vi "CH_LM ActiveX Control.vi"(0 "Communication Mode":T2, 1 "GPIB Board (0)":i16, 2 "MonitorStop Occurrence":refnum<k4>, 3 "error in (no error)":errorcluster) -> (5 "error out":errorcluster)   [LabVIEW 2017, in "CH_LM.lvlib"]
doc: "This VI is used to register ActiveX Event Callback VIs. Further more a Semaphore is created to make the CH_LM Transaction.vi thread save.\n\nAll important references, ActiveX Control, ActiveX Event Queue and Semaphore are stored in a Fuctional Global Variable for developer access.\n\n<B>Attention:</B> This VI has to be started first and must run all time to monitor event like Meter connected/Disconnected. The communication mode can be selected only once. LabVIEW must be restarted to select another communication mode.\n\n<B>Communication Mode</B> (an enumeration of USB, GPIB, RS232, or None)\nRead/write if no communication channels are open. \nRead only if one or more communication channels are open. \nSpecifies the communication mode. The uninitialized setting will be None. Until this property is set to something other than None:\n\" No events will fire\n\" No I/O activity will take place\n\" The SerialNumber property will return an empty string for any meter index\n\" The SendCommandOrQuery, ConnectToMeter, and DisconnectFromMeter methods will do nothing and return false for any meter index or string argument\n\" The GetNextString method will return an empty string for any meter index"
uses:
  CH_LM.lvlib
  CH_LM Communication Mode.ctl
  _CH_LM/CH_LM Event Cluster.ctl
  _CH_LM/CH_LM Action Enumeration.ctl
  <vilib>/Utility/error.llb/DialogType.ctl
panel:
  out "CH_LM Event Cluster":T1
  in  "CH_LM Event Cluster":T1
  in  "stop":bool
  in  "LM ActiveX Control":refnum<k7>(container)
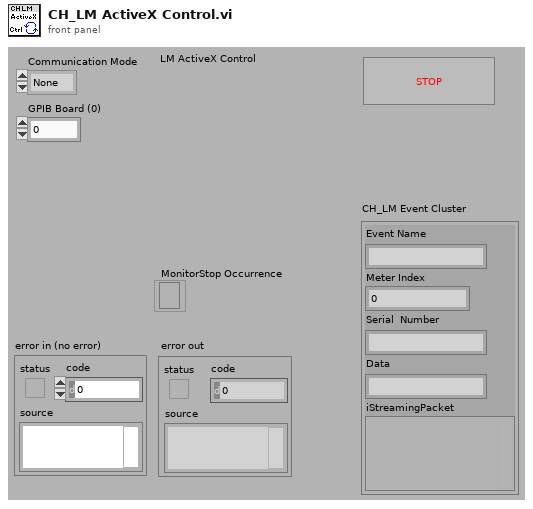
[diagram p1: front panel]
types:
  T1 = typedef "CH_LM.lvlib/CH_LM Event Cluster.ctl" = cluster{"Event Name":string, "Meter Index":i32, "Serial  Number":string, "Data":string, "iStreamingPacket":variant}
  T2 = typedef "CH_LM.lvlib/CH_LM Communication Mode.ctl" = enum16{"None", "USB", "GPIB", "RS232"}
  T3 = typedef "CH_LM.lvlib/CH_LM Action Enumeration.ctl" = enum16{"add", "read", "read by serial", "set", "remove", "delete", "Clear Shift-Register", ""}
  T4 = typedef "Semaphore RefNum" = refnum<k1>
  T5 = typedef "DialogType.ctl" = u16
  T6 = typedef "CH_LM Event Cluster.ctl" = cluster{"Event Name":string, "Meter Index":i32, "Serial  Number":string, "Data":string, "iStreamingPacket":variant}
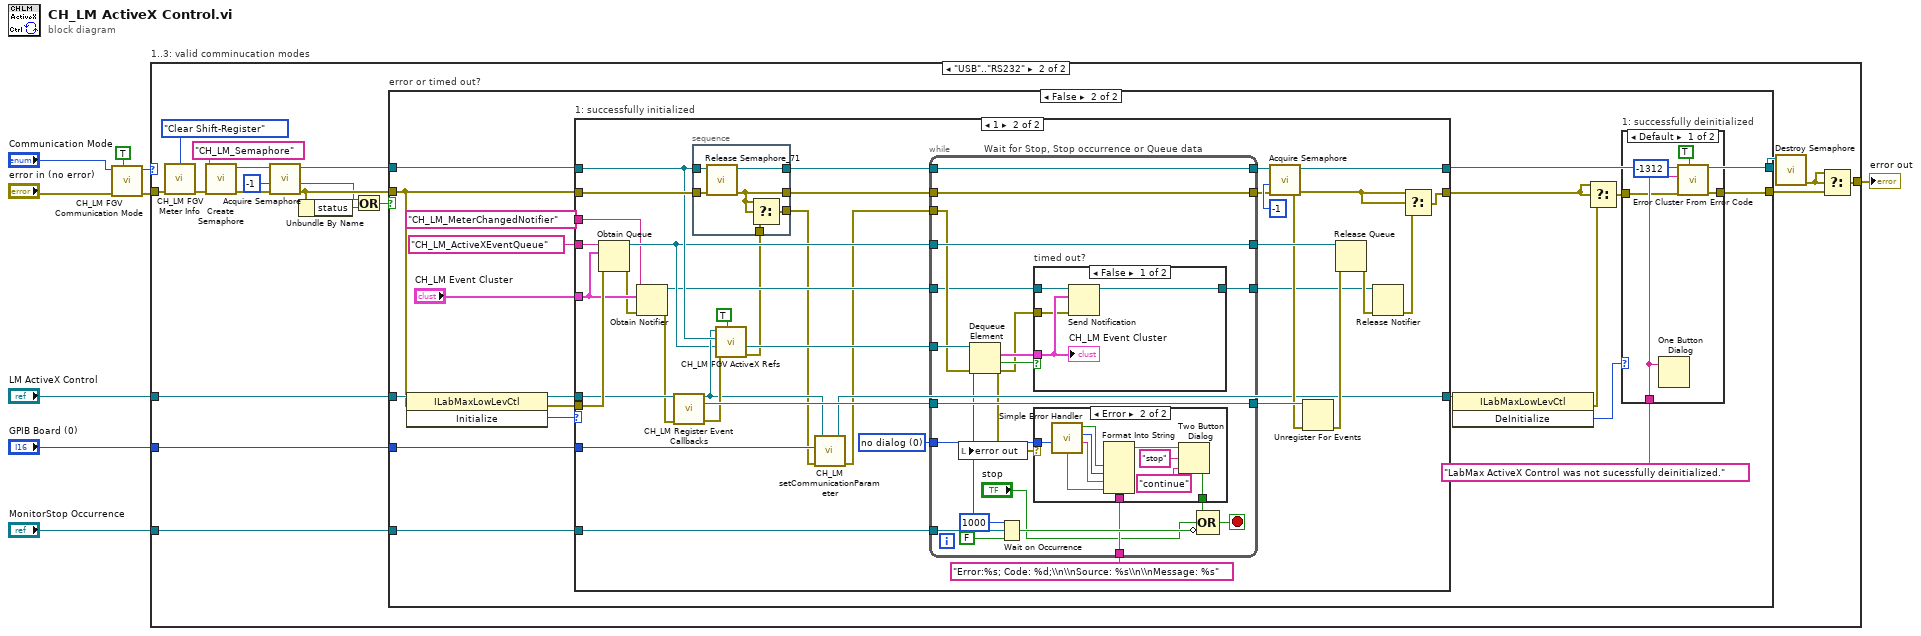
[diagram p0: block diagram]
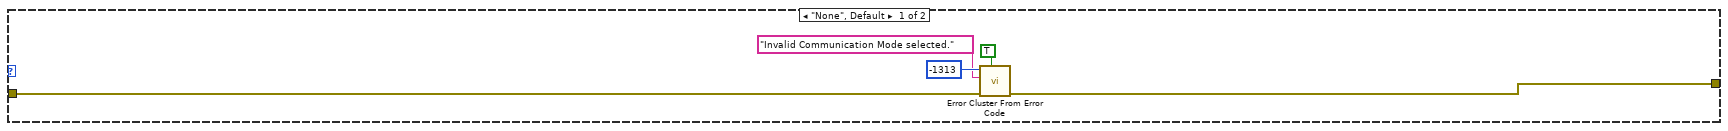
[diagram p2: hidden frame]
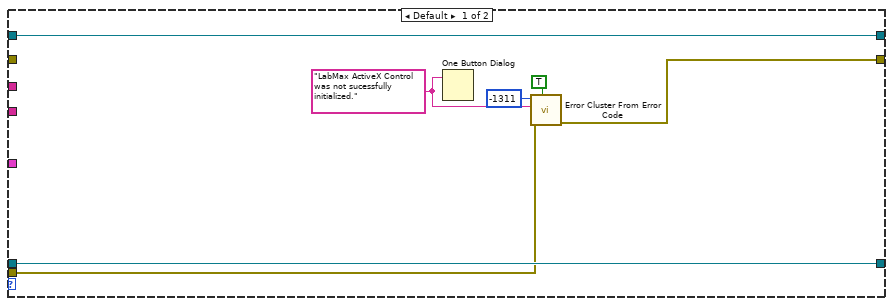
[diagram p5: hidden frame]
diagram:
  n1 = call "CH_LM FGV Communication Mode.vi"("set? (False)"=TRUE, "error in (no error)"="error in (no error)", "Communication Mode"="Communication Mode") -> ("error out"=w6:errorcluster, "Communication Mode"=w2:T2)  [unwired: 4 out]
  n2 = case "1..3: valid comminucation modes" shown="\"USB\"..\"RS232\"" w2 {
    tunnel: "MonitorStop Occurrence" -> [_ w33]
    tunnel: "LM ActiveX Control" -> [_ w25]
    tunnel: w6 -> [w14 w24]
    tunnel: [w10 w16] -> w7
    tunnel: "GPIB Board (0)" -> [_ w18]
    frame "None", Default {
      n3 = call <vilib>:"Error Cluster From Error Code.vi"("show call chain? (False)"=TRUE, "error in (no error)"=w14, "error message (\"\")"="Invalid Communication Mode selected." ("error message (\"\")"), "error code (0)"=-1313) -> ("error out"=w10:errorcluster)  [unwired: 5 out]
    }
    frame "USB".."RS232" {
      n4 = call "CH_LM FGV Meter Info.vi"("Action (read)"=CH_LM_Action_Enumeration."Clear Shift-Register", "error in (no error)"=w24) -> ("error out"=w32:errorcluster)  [unwired: 3 in, 10 out]
      n5 = call <vilib>:"Create Semaphore.vi"("error in (no error)"=w32, "name (unnamed)"="CH_LM_Semaphore" ("Rsrc Name")) -> ("error out"=w30:errorcluster, "semaphore"=w29:T4)  [unwired: 1 in, 3 out]
      n6 = call <vilib>:"Acquire Semaphore.vi"("error in (no error)"=w30, "ms timeout (-1)"=-1, "semaphore"=w29) -> ("error out"=w23:errorcluster, "timed out"=w21:bool, "semaphore out"=w26:T4)  [unwired: 2 out]
      n7 = Unbundle By Name(w23) -> ("status"=w22:bool)
      n8 = Or(x=w21, y=w22) -> (x .or. y?=w20:bool)
      n9 = case "error or timed out?" shown="False" w20 {
        tunnel: [w35 w39] -> w15
        tunnel: w33 -> [_ w54]
        tunnel: w25 -> [_ w52]
        tunnel: w23 -> [w35 w45]
        tunnel: w26 -> [w34 w53]
        tunnel: [w34 w49] -> w19
        tunnel: w18 -> [_ w47]
        frame True {
        }
        frame False {
          n10 = invoke class="ILabMaxLowLevCtl" method="Initialize"(reference=w52, error in=w45) -> (reference out=w51:refnum<k7>, error out=w48:errorcluster, "Initialize"=w50:i16)  [unwired: 1 in]
          n11 = case "1: successfully initialized" shown="1" w50 {
            tunnel: [w64 w105] -> w41
            tunnel: w54 -> [_ w98]
            tunnel: [w63 w82] -> w46
            tunnel: w45 -> [_ w89]
            tunnel: w53 -> [w62 w88]
            tunnel: w51 -> [w63 w81]
            tunnel: [w62 w86] -> w49
            tunnel: w48 -> [w61 w84]
            tunnel: w47 -> [_ w85]
            tunnel: "CH_LM_ActiveXEventQueue" ("Rsrc Name") -> [_ w80]
            tunnel: "CH_LM Event Cluster" -> [_ w77]
            tunnel: "CH_LM_MeterChangedNotifier" ("Rsrc Name") -> [_ w78]
            frame Default {
              w65 = "LabMax ActiveX Control was not sucessfully initialized." ("message")
              n12 = One Button Dialog(message=w65) -> ()  [unwired: 2 out]
              n13 = call <vilib>:"Error Cluster From Error Code.vi"("show call chain? (False)"=TRUE, "error in (no error)"=w61, "error message (\"\")"=w65, "error code (0)"=-1311) -> ("error out"=w64:errorcluster)  [unwired: 5 out]
            }
            frame 1 {
              w91 = T5 0 items=["no dialog", "OK message", "continue or stop message", "OK message + warnings", "continue/stop + warnings"] ("type of dialog (OK msg:1)")
              n14 = Obtain Queue(name (unnamed)=w80, element data type=w77, error in (no error)=w84) -> (queue out=w79:refnum<queue>, error out=w76:errorcluster)  [unwired: 2 in, 1 out]
              n15 = Obtain Notifier(name (unnamed)=w78, notification data type=w77, error in (no error)=w76) -> (notifier out=w74:refnum<notifier>, error out=w75:errorcluster)  [unwired: 1 in, 1 out]
              n16 = call "CH_LM Register Event Callbacks.vi"("CH_LM ActiveX Ref."=w81, "error in (no error)"=w75) -> ("dup CH_LM ActiveX Ref."=w83:refnum<k7>, "Event Callback refnum"=w97:refnum<k27>, "error out"=w90:errorcluster)  [unwired: 11 out]
              n17 = call "CH_LM FGV ActiveX Refs.vi"("set? (False)"=TRUE, "error in (no error)"=w90, "CH_LM Event queue"=w79, "CH_LM semaphore"=w88, "CH_LM ActiveX Ref."=w83) -> ("error out"=w70:errorcluster, "CH_LM Event queue"=w95:refnum<queue>)  [unwired: 2 out]
              n18 = stacked-sequence {
                tunnel: [w111] -> w102
                tunnel: [w108] -> w68
                tunnel: w88 -> [w110]
                tunnel: w89 -> [w109]
                tunnel: w70 -> [w107]
                tunnel: [w106] -> w92
                frame #0 {
                  n19 = call <vilib>:"Release Semaphore_71.vi"("error in (no error)"=w109, "semaphore"=w110) -> ("error out"=w106:errorcluster, "semaphore out"=w111:T4)  [unwired: 4 out]
                  n20 = Select(t=w106, s=w106, f=w107) -> (s? t:f=w108:errorcluster)
                }
              }
              n21 = call "CH_LM setCommunicationParameter.vi"("error in (no error)"=w68, "GPIB Board (0)"=w85, "CH_LM ActiveX Ref."=w83) -> ("error out"=w69:errorcluster, "dup CH_LM ActiveX Ref."=w82:refnum<k7>)  [unwired: 2 in, 1 out]
              n22 = while "Wait for Stop, Stop occurrence or Queue data" {
                tunnel: w102 -> [w129]
                tunnel: w79 -> [w130]
                tunnel: w97 -> [w131]
                tunnel: [w131] -> w101
                tunnel: [w130] -> w100
                tunnel: [w129] -> w99
                tunnel: w98 -> [w128]
                tunnel: w95 -> [w124]
                tunnel: w69 -> [w121]
                tunnel: "Error:%s; Code: %d;\\n\\nSource: %s\\n\\nMessage: %s" ("format string") -> [w118]
                tunnel: [w117] -> w93
                tunnel: w92 -> [w117]
                tunnel: w91 -> [w116]
                tunnel: w74 -> [w114]
                tunnel: [w112] -> w71
                stop <- w125 stop-if-true
                w123 = 1000 ("ms timeout (-1)")
                n23 = Dequeue Element(queue=w124, timeout in ms (-1)=w123, error in (no error)=w121) -> (element=w122:T6, timed out?=w120:bool, error out=w113:errorcluster)  [unwired: 1 out]
                n24 = local write "error out"(w113) -> ()
                n25 = Wait on Occurrence(1:FALSE ("ignore previous (T)"), 2:w128, 3:w123) -> (0:w126:bool)
                n26 = case "timed out?" shown="False" w120 {
                  tunnel: w122 -> [w144 _]
                  tunnel: w114 -> [w145 w146]
                  tunnel: w113 -> [w143 _]
                  tunnel: [w142 w146] -> w112
                  frame False {
                    n27 = Send Notification(notification=w144, notifier=w145, error in (no error)=w143) -> (notifier out=w142:refnum<notifier>)  [unwired: 1 out]
                    "CH_LM Event Cluster" <- w144
                  }
                  frame True {
                  }
                }
                n28 = case shown="Error" w113 {
                  tunnel: [_ w136] -> w119
                  tunnel: w118 -> [_ w135]
                  tunnel: w116 -> [_ w133]
                  frame No Error {
                  }
                  frame Error {
                    n29 = call <vilib>:"Simple Error Handler.vi"("type of dialog (OK msg:1)"=w133) -> ("error?"=w141:bool, "code out"=w140:i32, "source out"=w139:string, "message"=w138:string)  [unwired: 1 in, 4 out]
                    n30 = Format Into String(format string=w135, w141, w140, w139, w138) -> (resulting string=w137:string)  [unwired: 2 in, 1 out]
                    n31 = Two Button Dialog(message=w137, 1:"continue" ("F button name (\"Cancel\")"), 2:"stop" ("T button name (\"OK\")")) -> (T button?=w136:bool)
                  }
                }
                n32 = Compound Arithmetic op=OR(w119, "stop", invert w126) -> (w125:bool)
              }
              n33 = call <vilib>:"Acquire Semaphore.vi"("error in (no error)"=w93, "ms timeout (-1)"=-1, "semaphore"=w99) -> ("error out"=w87:errorcluster, "semaphore out"=w86:T4)  [unwired: 3 out]
              n34 = Unregister For Events(event registration refnum=w101, error in=w87) -> (error out=w104:errorcluster)
              n35 = Release Queue(queue=w100, error in (no error)=w104) -> (error out=w73:errorcluster)  [unwired: 3 out]
              n36 = Release Notifier(notifier=w71, error in (no error)=w73) -> (error out=w72:errorcluster)  [unwired: 3 out]
              n37 = Select(t=w87, s=w87, f=w72) -> (s? t:f=w105:errorcluster)
            }
          }
          n38 = invoke class="ILabMaxLowLevCtl" method="DeInitialize"(reference=w46) -> (error out=w42:errorcluster, "DeInitialize"=w43:i16)  [unwired: 2 in, 1 out]
          n39 = Select(t=w41, s=w41, f=w42) -> (s? t:f=w40:errorcluster)
          n40 = case "1: successfully deinitialized" shown="Default" w43 {
            tunnel: "LabMax ActiveX Control was not sucessfully deinitialized." ("message") -> [w57 _]
            tunnel: [w56 w60] -> w39
            tunnel: w40 -> [w55 w60]
            frame Default {
              n41 = One Button Dialog(message=w57) -> ()  [unwired: 2 out]
              n42 = call <vilib>:"Error Cluster From Error Code.vi"("show call chain? (False)"=TRUE, "error in (no error)"=w55, "error message (\"\")"=w57, "error code (0)"=-1312) -> ("error out"=w56:errorcluster)  [unwired: 5 out]
            }
            frame 1 {
            }
          }
        }
      }
      n43 = call <vilib>:"Destroy Semaphore.vi"("semaphore"=w19) -> ("error out"=w17:errorcluster)  [unwired: 1 in, 5 out]
      n44 = Select(t=w17, s=w17, f=w15) -> (s? t:f=w16:errorcluster)
    }
  }
  "error out" <- w7
